vi "Configure Reference Oscillator Auto Source.vi"(8 "error in (no error)":errorcluster, 10 "Auto Source (T:Enable)":bool=TRUE, 11 "VISA resource name":refnum<visa-resource-name>) -> (0 "error out":errorcluster, 3 "VISA resource name out":refnum<visa-resource-name>)   [LabVIEW 2011, in "Agilent PSG MXG Series.lvlib"]
doc: "Configures the ability of the signal generator to automatically select between the internal and an external reference oscillator.\n\n<B>Notes:</B>\n(1) For E8241A, E8244A, E8251A, E8254A, this VI is <B>NOT</B> valid when the instrument installs <B>Option UNJ</B> (Reference).\n\n(2) For E8247C, E8257C, E8267C, this VI is <B>NOT</B> valid when the instrument installs <B>Option UNR</B> (Enhanced phase noise performance).\n\n(3) For E8257D, E8267D, this VI is <B>NOT</B> valid when the instrument installs <B>Option UNR</B> or <B>Option UNX</B> (Ultra-low phase noise performance)."
uses:
  Agilent PSG MXG Series.lvlib
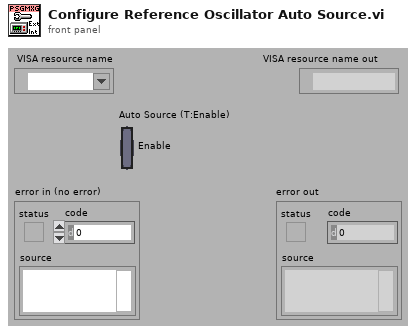
[diagram p1: front panel]
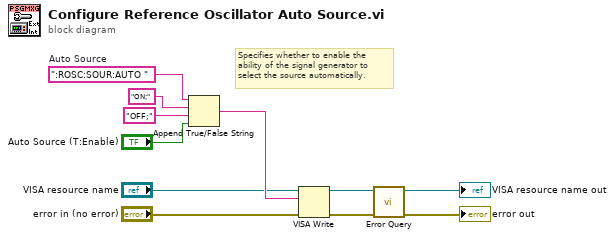
[diagram p0: block diagram]
diagram:
  w11 = ":ROSC:SOUR:AUTO "  # Auto Source
  # "Specifies whether to enable the\nability of the signal generator to\nselect the source automatically."
  n1 = Append True/False String(1:"Auto Source (T:Enable)", 2:"OFF;" ("false string"), 3:"ON;" ("true string"), 4:w11) -> (0:w7:string)
  n2 = VISA Write(VISA resource name="VISA resource name", write buffer=w7, error in (no error)="error in (no error)") -> (VISA resource name out=w6:refnum<visa-resource-name>, error out=w5:errorcluster)  [unwired: 1 out]
  n3 = call "Error Query.vi"("error in (no error)"=w5, "VISA resource name"=w6) -> ("error out"=→"error out":errorcluster, "VISA resource name out"=→"VISA resource name out":refnum<visa-resource-name>)  [unwired: 6 in, 2 out]
